vi "Stiffness Jacobian Column Dataset.vi"(8 "error in (no error)":errorcluster, 9 "Jacobian Stiffness Column In":T3, 10 "LBCB Number":T1, 11 "DAO Actions":T2) -> (0 "error out":errorcluster, 1 "Jacobian Stiffness Column Out":T3)   [LabVIEW 2009]
uses:
  Jacobian Stiffness Column.ctl
  Jacobian Stiffness Column Id.ctl
  Data Access Objects/Metadata/DAO Actions.ctl
  Data Access Objects/Metadata/LBCB Number.ctl
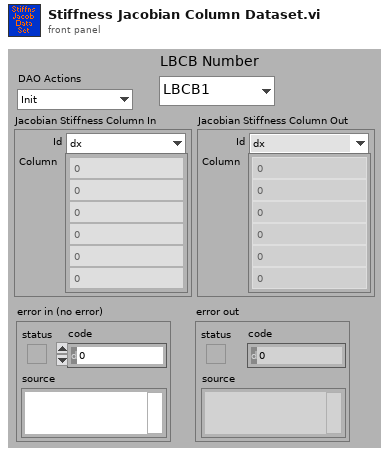
[diagram p1: front panel]
types:
  T1 = typedef "LBCB Number.ctl" = enum16{"LBCB1", "LBCB2"}
  T2 = typedef "DAO Actions.ctl" = enum16{"Init", "Get", "Set"}
  T3 = typedef "Jacobian Stiffness Column.ctl" = cluster{"Id":T4, "Column":dbl[]}
  T4 = typedef "Jacobian Stiffness Column Id.ctl" = enum16{"dx", "dy", "dz", "dRx", "dRy", "dRz"}
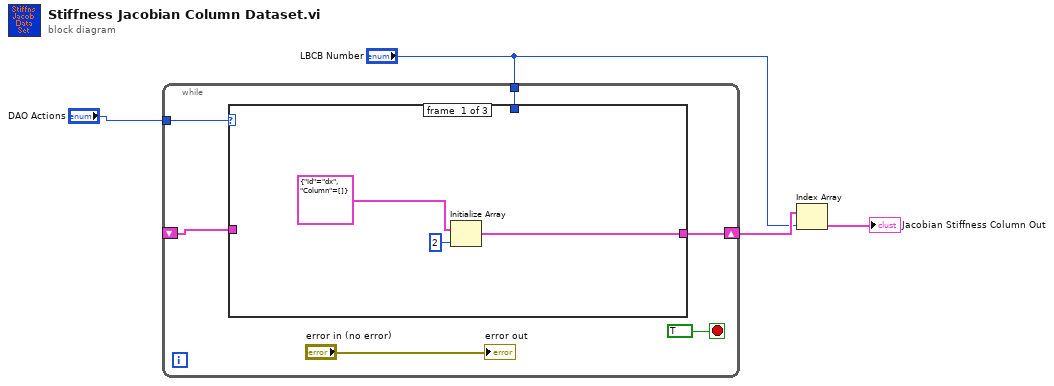
[diagram p0: block diagram]
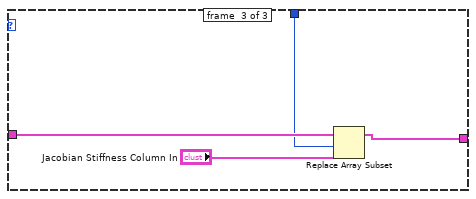
[diagram p3: hidden frame]
diagram:
  n1 = while {
    tunnel: "DAO Actions" -> [w9]
    shift-right: [w8] -> w2
    shift-left: _ -> [w7]
    tunnel: "LBCB Number" -> [w6]
    stop <- TRUE stop-if-true
    n2 = case shown="\"Get\"" w9 {
      tunnel: [w11 w14 w17] -> w8
      tunnel: w7 -> [_ w14 w18]
      tunnel: w6 -> [_ _ w15]
      frame #0 {
        n3 = Initialize Array(T3 {"Id"=enum."dx", "Column"=[]} ("Jacobian Stiffness Column In"), 2 ("dimension size")) -> (w11:T3[])
      }
      frame #1 {
      }
      frame #2 {
        n4 = Replace Array Subset(array=w18, new element="Jacobian Stiffness Column In", index=w15) -> (w17:T3[])
      }
    }
    "error out" <- "error in (no error)"
  }
  n5 = Index Array(array=w2, index="LBCB Number") -> (element=→"Jacobian Stiffness Column Out":T3)
